vi "Write Repeat Delay.vi"(8 "error in (no error)":errorcluster, 10 "Repeat Delay":i32, 11 "Content in":refnum<class "Content.lvclass">) -> (0 "error out":errorcluster, 3 "Content out":refnum<class "Content.lvclass">)   [LabVIEW 2026, in "LED Matrix.lvlib" / "Content.lvclass"]
uses:
  Content.lvclass
  Content.lvclass/Content.ctl
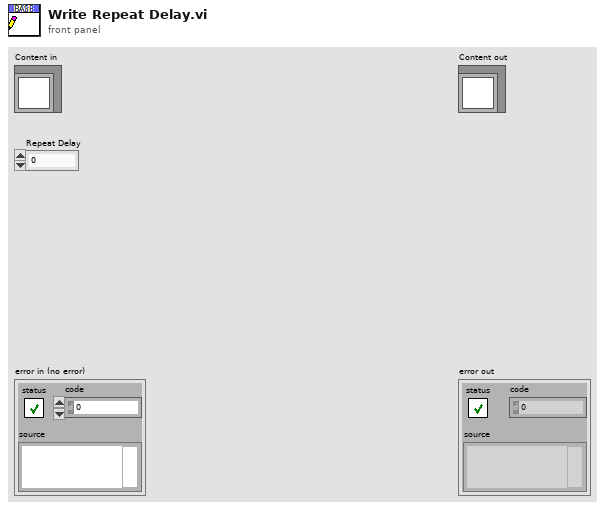
[diagram p1: front panel]
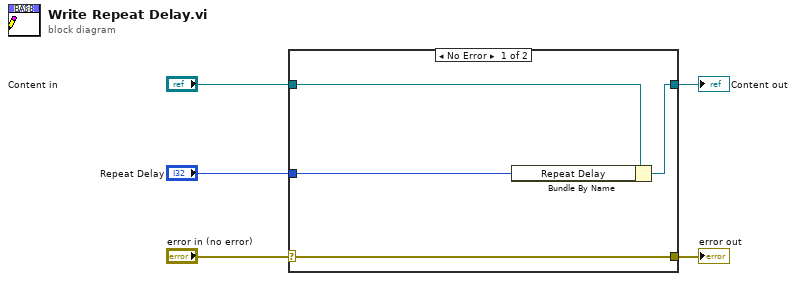
[diagram p0: block diagram]
diagram:
  n1 = case shown="No Error" "error in (no error)" {
    selector: "error in (no error)" -> [w9 w10]
    tunnel: [w9 w10] -> w4
    tunnel: [w7 w11] -> w2
    tunnel: "Content in" -> [w8 w11]
    tunnel: "Repeat Delay" -> [w6 _]
    frame No Error {
      n2 = Bundle By Name(cluster=w8, "Repeat Delay"=w6) -> (w7:refnum<class "Content.lvclass">)
    }
    frame Error {
    }
  }
  "error out" <- w4
  "Content out" <- w2
